vi "Get Client fp.vi"(8 "error in":errorcluster, 10 "Client Name":string, 11 "Client Manager in":refnum<class "Client Manager.lvclass">) -> (0 "error out":errorcluster, 2 "Client fp":path, 3 "Client Manager out":refnum<class "Client Manager.lvclass">)   [LabVIEW 2014, in "Client Manager.lvclass"]
uses:
  Client Manager.lvclass
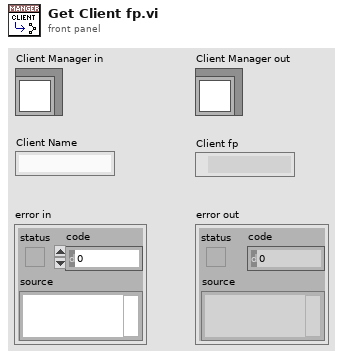
[diagram p1: front panel]
types:
  T1 = cluster{"Client Name":string, "Client fp":path}[]
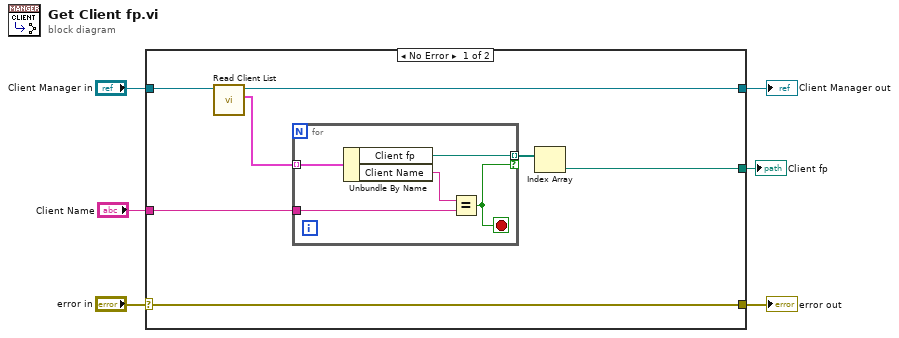
[diagram p0: block diagram]
diagram:
  n1 = case shown="No Error" "error in" {
    selector: "error in" -> [w12 w20]
    tunnel: [w12 w20] -> w5
    tunnel: [w11 w19] -> w3
    tunnel: "Client Manager in" -> [w13 w19]
    tunnel: "Client Name" -> [w9 _]
    tunnel: [w7 _] -> w1
    frame No Error {
      n2 = call-dynamic "Read Client List.vi"("Client Manager in"=w13) -> ("Client List"=w10:T1, "Client Manager out"=w11:refnum<class "Client Manager.lvclass">)  [unwired: 8 in, 1 out]
      n3 = for {
        tunnel: w10 -> [w18] mode=indexing
        tunnel: [w17] -> w8 mode=indexing if=w14
        tunnel: w9 -> [w16]
        stop <- w14 stop-if-true
        n4 = Unbundle By Name(w18) -> ("Client fp"=w17:path, "Client Name"=w15:string)
        n5 = Equal?(x=w15, y=w16) -> (x = y?=w14:bool)
      }
      n6 = Index Array(array=w8) -> (element=w7:path)  [unwired: 1 in]
    }
    frame Error {
    }
  }
  "error out" <- w5
  "Client Manager out" <- w3
  "Client fp" <- w1
